vi "MiniWheel Control Code.vi"() -> ()   [LabVIEW 2016]
uses:
  Instance           1 16Saved   example1 .vi
  <userlib>/dynamixel/dynamixel.lvlib
panel:
  in  "stop 2":bool
  in  "Wheel Dynamixel ID":i32=1
  in  "Goal Omega":u16=512 max=1023 step=1
  in  "Rotator Dynamixel ID":i32=1
  in  "Com Port":i32=3
  in  "Baud Rate":i32=1
  in  "stop":bool
  out "Present Position":u16(slide) max=1023 scale=0.0..1023.0
  in  "Goal position":u16=512 max=1023 step=1
  # "Motor Feedback"
  # "Initialization"
  # "Parameters"
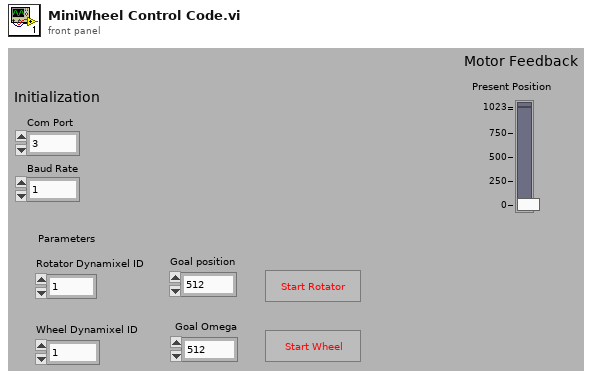
[diagram p1: front panel]
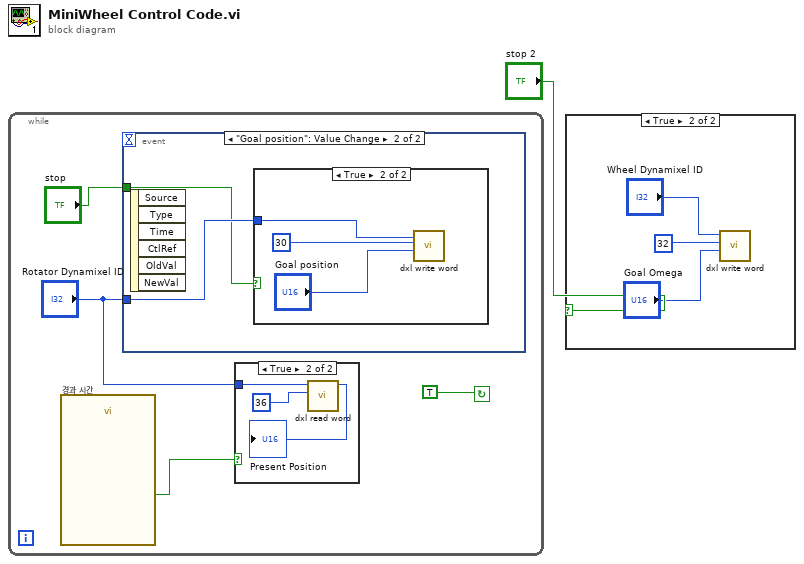
[diagram p0: block diagram]
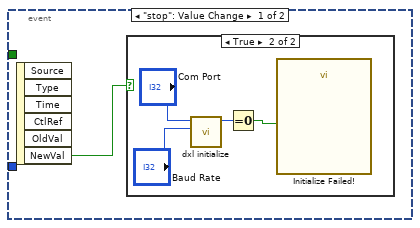
[diagram p4: hidden frame]
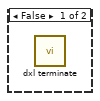
[diagram p5: hidden frame]
diagram:
  n1 = while {
    stop <- TRUE continue-if-true
    n2 = call "경과 시간"() -> ("Time has Elapsed"=w3:bool)  [unwired: 12 in, 7 out]
    n3 = event shown="[1] \"Goal position\": Value Change" {
      selector: _ -> [_ _]
      dyn-events: _ -> [_ _]
      timeout: _ -> [_ _]
      tunnel: "Rotator Dynamixel ID" -> [_ w15]
      tunnel: "stop" -> [_ w14]
      event "stop": Value Change {
        n4 = event-data() -> ("NewVal"=w9:bool)  [unwired: 1 in, 5 out]
        n5 = case shown="True" w9 {
          frame False {
            n6 = call <userlib>:"dxl terminate.vi"() -> ()  [unwired: 12 in]
          }
          frame True {
            n7 = call <userlib>:"dxl initialize.vi"("baudnum"="Baud Rate", "devIndex"="Com Port") -> ("function return"=w12:i32)  [unwired: 9 in]
            n8 = Equal To 0?(x=w12) -> (x = 0?=w13:bool)
            n9 = call "Initialize Failed!"("Enable"=w13) -> ()  [unwired: 9 in, 2 out]
          }
        }
      }
      event "Goal position": Value Change {
        n10 = event-data() -> ()  [unwired: 1 in, 6 out]
        n11 = case shown="True" w14 {
          tunnel: w15 -> [_ w18]
          frame False {
          }
          frame True {
            n12 = call <userlib>:"dxl write word.vi"("value"="Goal position", "address"=30, "id"=w18) -> ()  [unwired: 9 in]
          }
        }
      }
    }
    n13 = case shown="True" w3 {
      tunnel: "Rotator Dynamixel ID" -> [_ w7]
      frame False {
      }
      frame True {
        n14 = call <userlib>:"dxl read word.vi"("address"=36, "id"=w7) -> ("function return"=→"Present Position":i32)  [unwired: 9 in]
      }
    }
  }
  n15 = case shown="True" "stop 2" {
    frame False {
    }
    frame True {
      n16 = call <userlib>:"dxl write word.vi"("value"="Goal Omega", "address"=32, "id"="Wheel Dynamixel ID") -> ()  [unwired: 9 in]
    }
  }
